vi "SVPO RMS Level (1 Ch DBL Array) with IC.vi"(6 "restart averaging? (F)":bool, 8 "initial conditions":T1, 10 "sampling rate [Hz]":dbl=1.0, 11 "scaled signal [EU]":dbl[](array[numeric])) -> (0 "final conditions":T1, 3 "RMS level":dbl=nan, 4 "duration [s]":dbl)   [LabVIEW 2017, in "SoundVib_VibrationLevel.lvlib"]
doc: "Computes the root-mean-square (RMS) level of scaled time waveform signals and scaled array signals. <B>scaled signal [EU]</B> should have a zero DC component. You can attenuate the DC component with hardware AC-coupling filters and with software high-pass filters. Use this VI on embedded targets that have limited computational resources. Wire data to the <B>scaled signal [EU]</B> input to determine the polymorphic instance to use or manually select the instance."
uses:
  <vilib>/addons/Sound and Vibration/svt_Level/SoundVib_VibrationLevel.lvlib
  <vilib>/addons/_NISVFA/_Shared subVIs/Controls/svc_RMS Level State.ctl
  <vilib>/Analysis/baseanly.llb/Real Dot Product.vi
  <vilib>/Analysis/NI_AALBase.lvlib
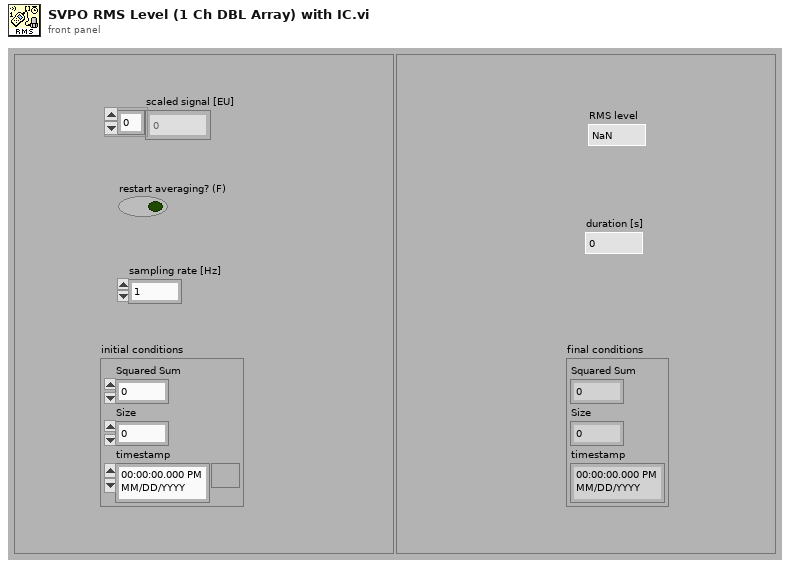
[diagram p1: front panel]
types:
  T1 = typedef "svc_RMS Level State.ctl" = cluster{"Squared Sum":dbl, "Size":u64, "timestamp":timestamp}
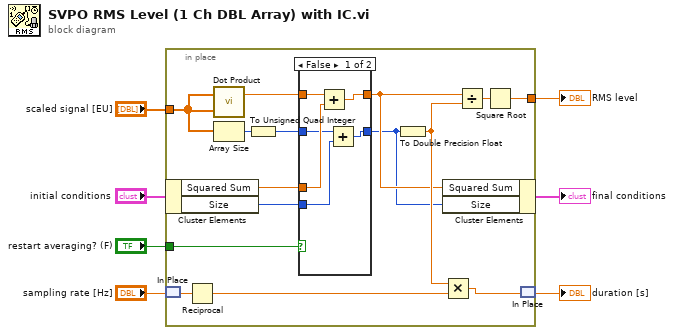
[diagram p0: block diagram]
diagram:
  n1 = in-place {
    in-place-border: "scaled signal [EU]" -> [w20]
    in-place-border: [w19] -> w6
    in-place-border: "restart averaging? (F)" -> [w18]
    n2 = in-place-cluster #1("initial conditions") -> ("Squared Sum"=w17:dbl, "Size"=w16:u64)
    n3 = in-place-match #2("sampling rate [Hz]") -> (w14:dbl)
    n4 = Reciprocal(x=w14) -> (1/x=w22:dbl)
    n5 = call-poly <vilib>:"Dot Product.vi"("Y Vector"=w20, "X Vector"=w20) -> ("X * Y"=w11:dbl)  [unwired: 1 out]
    n6 = Array Size(array=w20) -> (size(s)=w13:i32)
    n7 = To Unsigned Quad Integer(1:w13) -> (0:w9:u64)
    n8 = case shown="False" w18 {
      tunnel: [w26 w30] -> w10
      tunnel: w16 -> [w25 _]
      tunnel: w17 -> [w27 _]
      tunnel: w11 -> [w28 w30]
      tunnel: w9 -> [w24 w29]
      tunnel: [w23 w29] -> w8
      frame False {
        n9 = Add(x=w28, y=w27) -> (x+y=w26:dbl)
        n10 = Add(x=w24, y=w25) -> (x+y=w23:u64)
      }
      frame True {
      }
    }
    n11 = To Double Precision Float(number=w8) -> (double precision float=w12:dbl)
    n12 = in-place-cluster #1("Squared Sum"=w10, "Size"=w8) -> (→"final conditions":T1)
    n13 = Multiply(x=w12, y=w22) -> (x*y=w15:dbl)
    n14 = Divide(x=w10, y=w12) -> (x/y=w21:dbl)
    n15 = Square Root(x=w21) -> (sqrt(x)=w19:dbl)
    n16 = in-place-match #2(w15) -> (→"duration [s]":dbl)
  }
  "RMS level" <- w6
